vi "Brace_process_stream.vi"(8 "error in (no error)":errorcluster, 10 "Sensor Indicies":i32[](array[numeric]), 11 "Data Packet":string) -> (0 "error out":errorcluster, 1 "B xyz":dbl[][](array[numeric]), 3 "Time out":u32, 4 "Sensors (uT)":dbl[][](array[numeric]), 5 "Boolean":bool)   [LabVIEW 2018]
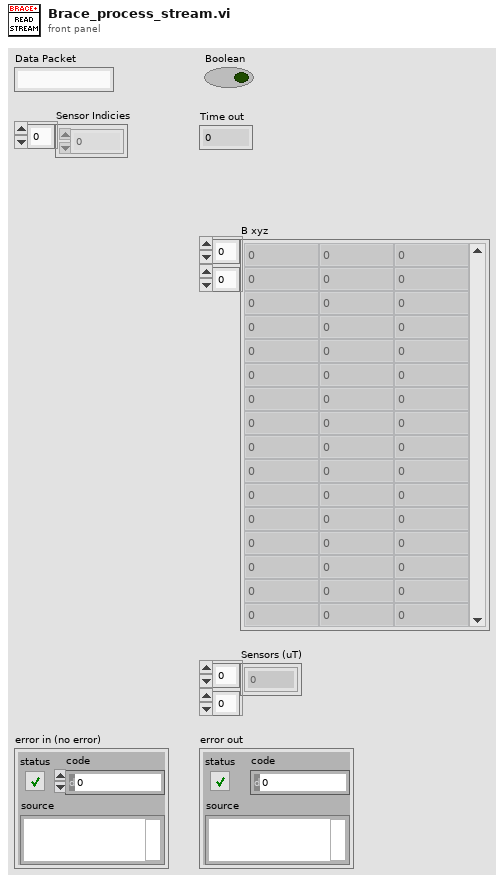
[diagram p1: front panel]
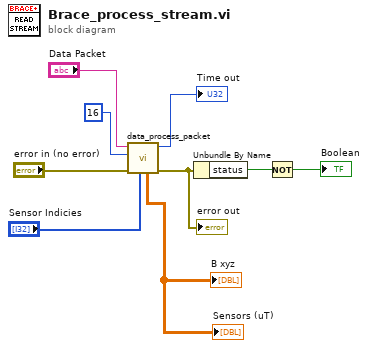
[diagram p0: block diagram]
diagram:
  n1 = call "data_process_packet.vi"("Sensor Lookup Indices"="Sensor Indicies", "error in (no error)"="error in (no error)", "No. Sensors"=16 ("No. Nodes"), "Binary Input Data"="Data Packet") -> ("error out"=w8:errorcluster, "Time"=→"Time out":u32, "Sensors (uT)"=→"B xyz" →"Sensors (uT)":dbl[][])  [unwired: 3 in, 2 out]
  "error out" <- w8
  n2 = Unbundle By Name(w8) -> ("status"=w1:bool)
  n3 = Not(x=w1) -> (.not. x?=→"Boolean":bool)
